vi "Brace_sys_stream.vi"(8 "error in (no error)":errorcluster, 9 "Packet Size (Bytes)":u32, 10 "Numeric":i32, 11 "VISA Refnum in":refnum<visa-resource-name>) -> (0 "error out":errorcluster, 2 "Data Out":string, 3 "VISA Refnum out":refnum<visa-resource-name>)   [LabVIEW 2018]
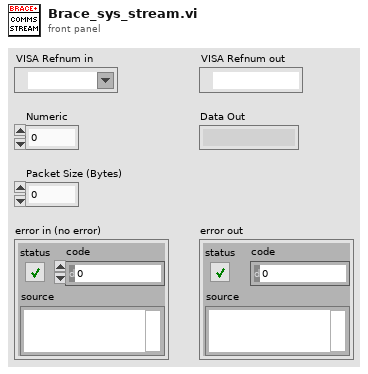
[diagram p1: front panel]
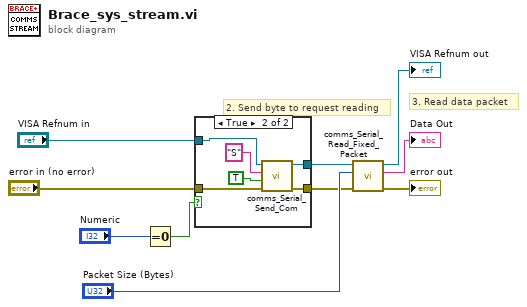
[diagram p0: block diagram]
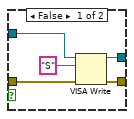
[diagram p2: hidden frame]
diagram:
  # "3. Read data packet"
  # "2. Send byte to request reading"
  n1 = Equal To 0?(x="Numeric") -> (x = 0?=w2:bool)
  n2 = case shown="True" w2 {
    tunnel: "VISA Refnum in" -> [w15 w21]
    tunnel: [w14 w19] -> w4
    tunnel: [w12 w18] -> w3
    tunnel: "error in (no error)" -> [w11 w16]
    frame False {
      n3 = VISA Write(VISA resource name=w15, write buffer="S", error in (no error)=w11) -> (VISA resource name out=w14:refnum<visa-resource-name>, error out=w12:errorcluster)  [unwired: 1 out]
    }
    frame True {
      n4 = call "comms_Serial_Send_Com.vi"("error in"=w16, "Buffer Clear?"=TRUE, "Command"="S", "VISA resource in"=w21) -> ("error out"=w18:errorcluster, "VISA resource Out"=w19:refnum<visa-resource-name>)  [unwired: 5 in, 1 out]
    }
  }
  n5 = call "comms_Serial_Read_Fixed_Packet.vi"("error in"=w3, "Packet Size (Bytes)"="Packet Size (Bytes)", "VISA resource in"=w4) -> ("error out"=→"error out":errorcluster, "Data Out"=→"Data Out":string, "VISA resource Out"=→"VISA Refnum out":refnum<visa-resource-name>)  [unwired: 4 in, 2 out]
